vi "KE622x -- Get Voltage Limit.vi"(0 "Resource In":refnum<visa-resource-name>, 1 "Check For SCPI Errors? (T)":bool=TRUE, 11 "error in (no error)":errorcluster) -> (4 "Resource Out (dupl)":refnum<visa-resource-name>, 8 "Voltage Limit (V) 2":T1=10.0 min=0.1 max=105.0 step=0.01 format="%.2p", 15 "error out":errorcluster)   [LabVIEW 2013, in "Keithly user program.lvlib"]
doc: "Returns the voltage limit (compliance) for the current source."
uses:
  Keithly user program.lvlib
  Typedefs/KE622x -- Voltage Limit.ctl
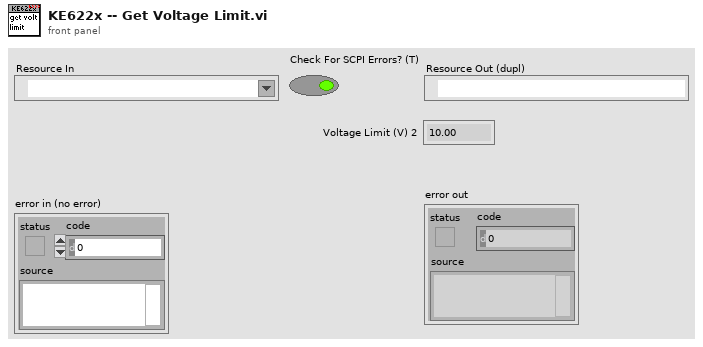
[diagram p1: front panel]
types:
  T1 = typedef "Keithly user program.lvlib/KE622x -- Voltage Limit.ctl" = dbl
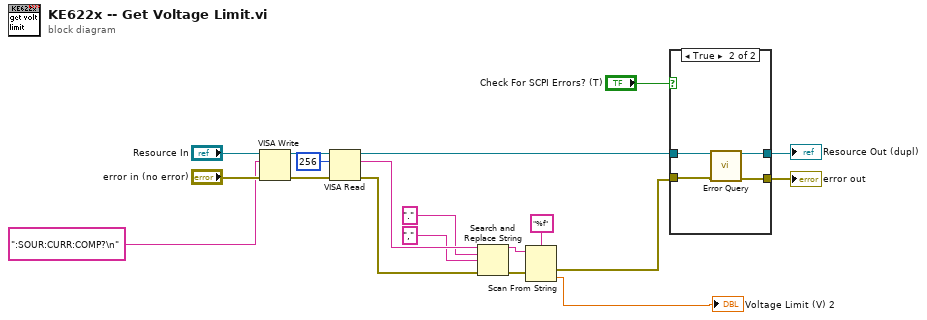
[diagram p0: block diagram]
diagram:
  n1 = VISA Write(VISA resource name="Resource In", write buffer=":SOUR:CURR:COMP?\n" ("format string"), error in (no error)="error in (no error)") -> (VISA resource name out=w13:refnum<visa-resource-name>, error out=w12:errorcluster)  [unwired: 1 out]
  n2 = VISA Read(VISA resource name=w13, byte count=u32 256, error in (no error)=w12) -> (VISA resource name out=w8:refnum<visa-resource-name>, read buffer=w5:string, error out=w6:errorcluster)  [unwired: 1 out]
  n3 = Search and Replace String(input string=w5, search string=".", replace string="," ("replace string (\"\")"), error in=w6) -> (result string=w2:string, error out=w7:errorcluster)  [unwired: 4 in, 2 out]
  n4 = Scan From String(format string="%f", input string=w2, error in=w7) -> (error out=w9:errorcluster, output 1=→"Voltage Limit (V) 2":T1)  [unwired: 2 in, 2 out]
  n5 = case shown="True" "Check For SCPI Errors? (T)" {
    tunnel: w8 -> [w21 w22]
    tunnel: w9 -> [w20 w23]
    tunnel: [w20 w24] -> w15
    tunnel: [w21 w25] -> w16
    frame False {
    }
    frame True {
      n6 = call "Error Query.vi"("VISA Resource In"=w22, "error in (no error)"=w23) -> ("VISA Resource Out (dupl)"=w25:refnum<visa-resource-name>, "error out"=w24:errorcluster)  [unwired: 10 in, 2 out]
    }
  }
  "Resource Out (dupl)" <- w16
  "error out" <- w15
